vi "Configuration 1.0 Initialize.vi"(8 "error in (no error)":errorcluster, 10 "dsf version":T2, 11 "dsf configuration json":string) -> (0 "error out":errorcluster, 3 "framework configuration 1.0":T1)   [LabVIEW 2017, in "DSF Core.lvlib" / "Configuration Session.lvclass"]
uses:
  Configuration Session.lvclass
  Typedefs/DSF Version Info.ctl
  DSF Core.lvlib
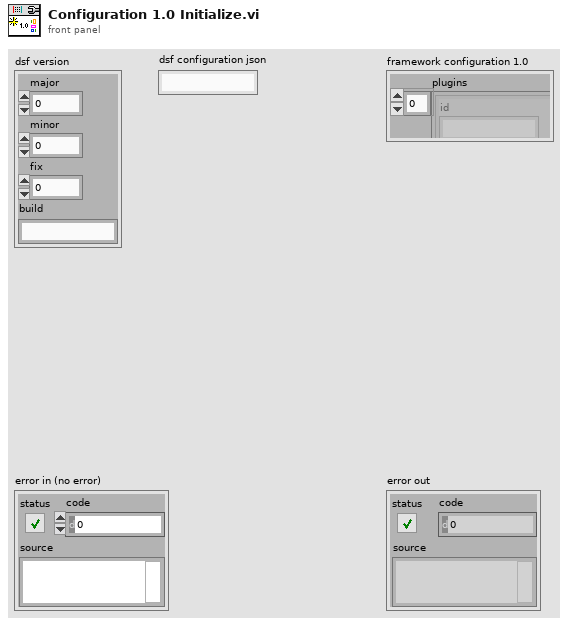
[diagram p1: front panel]
types:
  T1 = cluster{"plugins":cluster{"id":string, "values":cluster{"components":string[], "timing":cluster{"priority":u64, "decimation":u64, "offset":u64}, "group ids":string[], "settings id":string, "threads":cluster{"buffer converter settings":cluster{"key":string, "value":string}[], "transceiver settings":cluster{"key":string, "value":string}[], "custom settings":cluster{"key":string, "value":string}[], "processor":i32, "priority offset":i16}[]}}[], "groups":cluster{"id":string, "values":cluster{"direction":i32, "timing":cluster{"priority":u64, "decimation":u64, "offset":u64}, "transfer ids":string[], "settings id":string, "thread":i32, "timeout behavior":u8}}[], "transfers":cluster{"id":string, "values":cluster{"byte order":i32, "channel ids":string[], "settings id":string}}[], "channels":cluster{"id":string, "values":cluster{"string buffer offset":u64, "string data type":i32, "engine data type":i32, "settings id":string, "units":string}}[], "settings":cluster{"id":string, "values":cluster{"key":string, "value":string}[]}[]}
  T2 = typedef "DSF Core.lvlib/DSF Version Info.ctl" = cluster{"major":u32, "minor":u32, "fix":u32, "build":string}
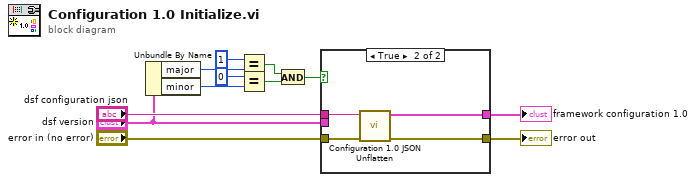
[diagram p0: block diagram]
diagram:
  n1 = Unbundle By Name("dsf version") -> ("major"=w9:u32, "minor"=w11:u32)
  n2 = Equal?(x=u32 1, y=w9) -> (x = y?=w5:bool)
  n3 = Equal?(x=u32 0, y=w11) -> (x = y?=w6:bool)
  n4 = And(x=w5, y=w6) -> (x .and. y?=w4:bool)
  n5 = case shown="True" w4 {
    tunnel: "error in (no error)" -> [w13 w14]
    tunnel: "dsf configuration json" -> [_ w17]
    tunnel: [_ w16] -> w1
    tunnel: [w13 w15] -> w10
    tunnel: "dsf version" -> [_ _]
    frame False {
      # "Unknown version."
    }
    frame True {
      n6 = call "Configuration 1.0 JSON Unflatten.vi"("error in (no error)"=w14, "dsf configuration json"=w17) -> ("error out"=w15:errorcluster, "framework configuration 1.0"=w16:T1)  [unwired: 7 in, 1 out]
    }
  }
  "error out" <- w10
  "framework configuration 1.0" <- w1
